vi "Wait for ReaderState.vi"(8 "error in (no error)":errorcluster, 9 "timeout (5000 ms)":i32=5000, 11 "Target WriterState (T-Running/F-Idle)":bool) -> (0 "error out":errorcluster, 3 "timeout?":bool)   [LabVIEW 2021, in "XNET-CAN-Signal-Logger.lvlib"]
uses:
  XNET-CAN-Signal-Logger.lvlib
  Global Variables.vi
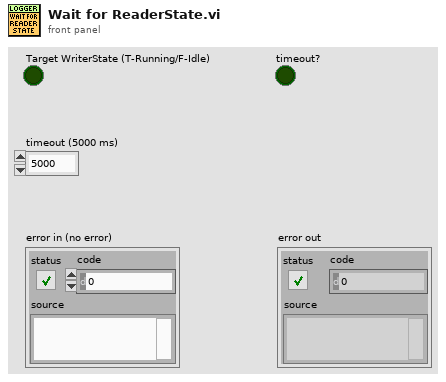
[diagram p1: front panel]
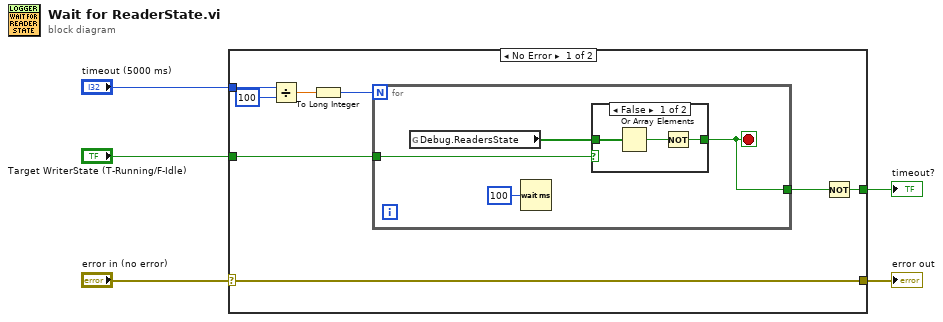
[diagram p0: block diagram]
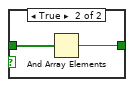
[diagram p2: hidden frame]
diagram:
  n1 = case shown="No Error" "error in (no error)" {
    selector: "error in (no error)" -> [w6 w23]
    tunnel: "Target WriterState (T-Running/F-Idle)" -> [w12 _]
    tunnel: [w11 _] -> w4
    tunnel: "timeout (5000 ms)" -> [w10 _]
    tunnel: [w6 w23] -> w2
    frame No Error {
      n2 = Divide(x=w10, y=100) -> (x/y=w9:dbl)
      n3 = To Long Integer(number=w9) -> (32bit integer=w7:i32)
      n4 = for {
        N: w7 -> [_]
        tunnel: [w15] -> w13
        tunnel: w12 -> [w14]
        stop <- w15 stop-if-true
        n5 = global read "Global Variables.vi" "Debug.ReadersState"() -> (w16:bool[])
        n6 = Wait (ms)(milliseconds to wait=u32 100) -> ()  [unwired: 1 out]
        n7 = case shown="False" w14 {
          tunnel: w16 -> [w20 w22]
          tunnel: [w19 w21] -> w15
          frame False {
            n8 = Or Array Elements(Boolean array=w20) -> (logical OR=w18:bool)
            n9 = Not(x=w18) -> (.not. x?=w19:bool)
          }
          frame True {
            n10 = And Array Elements(Boolean array=w22) -> (logical AND=w21:bool)
          }
        }
      }
      n11 = Not(x=w13) -> (.not. x?=w11:bool)
    }
    frame Error {
    }
  }
  "timeout?" <- w4
  "error out" <- w2
